vi "Two BTN User Message XL.vi"(4 "Option 2 (\"Stop\")":string="Stop", 6 "Option 1 (\"OK\")":string="OK", 10 "Message":string) -> (1 "Ok?":bool)   [LabVIEW 2021]
panel:
  in  "Stop":bool
  in  "OK":bool
  in  "Title":string
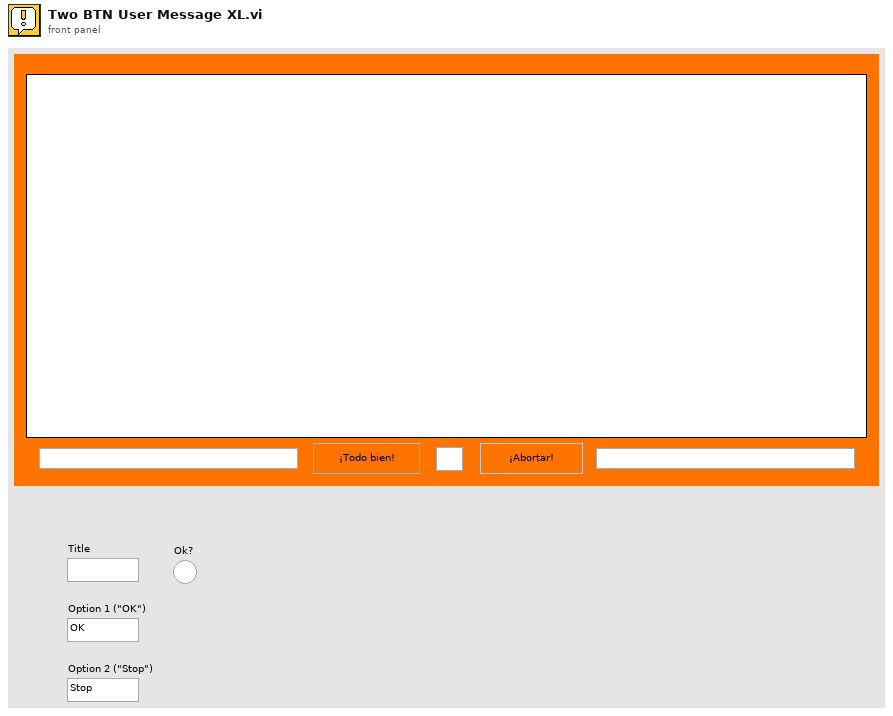
[diagram p1: front panel]
types:
  T1 = cluster{"accent s color":u32, "accent s color":u32}
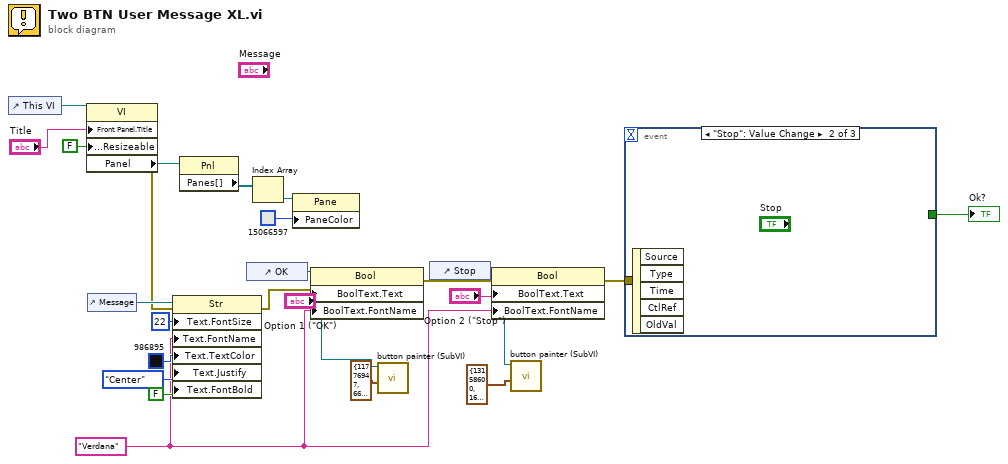
[diagram p0: block diagram]
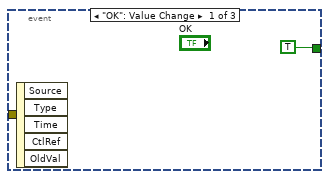
[diagram p2: hidden frame]
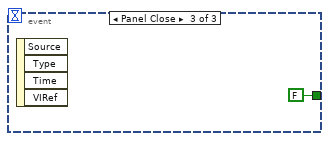
[diagram p3: hidden frame]
diagram:
  w1 = "Verdana" ("Text.Font:Name")
  n1 = control-ref of="This VI"() -> (w19:refnum<vi>)
  n2 = property class="VI"(reference=w19, "Front Panel.Title"="Title", "Front Panel.Resizeable"=FALSE ("Front Panel Window:Resizable")) -> (error out=w17:errorcluster, "Panel"=w15:refnum<vi>)  [unwired: 1 in, 1 out]
  n3 = control-ref of="Message"() -> (w24:refnum<vi>)
  n4 = property on="Property Node" class="Str"(reference=w24, error in=w17, "Text.FontSize"=u32 22 ("Text.Font:Size"), "Text.FontName"=w1, "Text.TextColor"=u32 986895 ("Text.Text Colors:Text Color"), "Text.Justify"=enum16{"Left", "Center", "Right"}."Center" ("Text.Justification"), "Text.FontBold"=FALSE ("Text.Font:Bold")) -> (error out=w9:errorcluster)  [unwired: 1 out]
  n5 = property class="Pnl"(reference=w15) -> ("Panes[]"=w14:refnum<vi>[])  [unwired: 1 in, 2 out]
  n6 = control-ref of="OK"() -> (w5:refnum<vi>)
  n7 = Index Array(array=w14) -> (element=w13:refnum<vi>)  [unwired: 1 in]
  n8 = property class="Pane"(reference=w13, "PaneColor"=u32 15066597 ("Pane Color")) -> ()  [unwired: 1 in, 2 out]
  n9 = property on="Property Node" class="Bool"(reference=w5, error in=w9, "BoolText.Text"="Option 1 (\"OK\")", "BoolText.FontName"=w1) -> (error out=w8:errorcluster)  [unwired: 1 out]
  n10 = call "button painter (SubVI).vi"("Off state"=cluster{"accent color":u32, "accent color":u32} {"accent color"=11776947, "accent color"=6618880}, "Button ref in"=w5) -> ()  [unwired: 10 in]
  n11 = control-ref of="Stop"() -> (w3:refnum<vi>)
  n12 = property on="Property Node" class="Bool"(reference=w3, error in=w8, "BoolText.Text"="Option 2 (\"Stop\")", "BoolText.FontName"=w1) -> (error out=w7:errorcluster)  [unwired: 1 out]
  n13 = call "button painter (SubVI).vi"("Off state"=T1 {"accent s color"=13158600, "accent s color"=16719363} ("On state"), "Button ref in"=w3) -> ()  [unwired: 10 in]
  n14 = event shown="[1] \"Stop\": Value Change" {
    selector: _ -> [_ _ _]
    dyn-events: _ -> [_ _ _]
    timeout: _ -> [_ _ _]
    tunnel: [TRUE _ FALSE] -> w20
    tunnel: w7 -> [_ _ _]
    event "OK": Value Change {
      n15 = event-data() -> ()  [unwired: 6 out]
    }
    event "Stop": Value Change {
      n16 = event-data() -> ()  [unwired: 6 out]
    }
    event Panel Close {
      n17 = event-data() -> ()  [unwired: 5 out]
    }
  }
  "Ok?" <- w20
